vi "Text.vi"(4 "text color(black)":u32(colorbox), 5 "[user-specified font]":T1={"Font Name:"="", "Size"=12, "Strikeout?"=FALSE, "Italic?"=FALSE, "Underline?"=FALSE, "Outline?"=FALSE, "Shadow?"=FALSE, "Bold?"=FALSE}, 6 "alignment(left, top)":T2, 7 "text":string, 8 "error in (no error)":errorcluster, 9 "origin":cluster{"x":i16, "y":i16}, 10 "picture":picture) -> (0 "error out":errorcluster, 2 "new picture":picture)   [LabVIEW 2020, in "lv_icon.lvlib"]
doc: "Add text to a given glyph."
uses:
  <vilib>/LabVIEW Icon API/lv_icon/lv_icon.lvlib
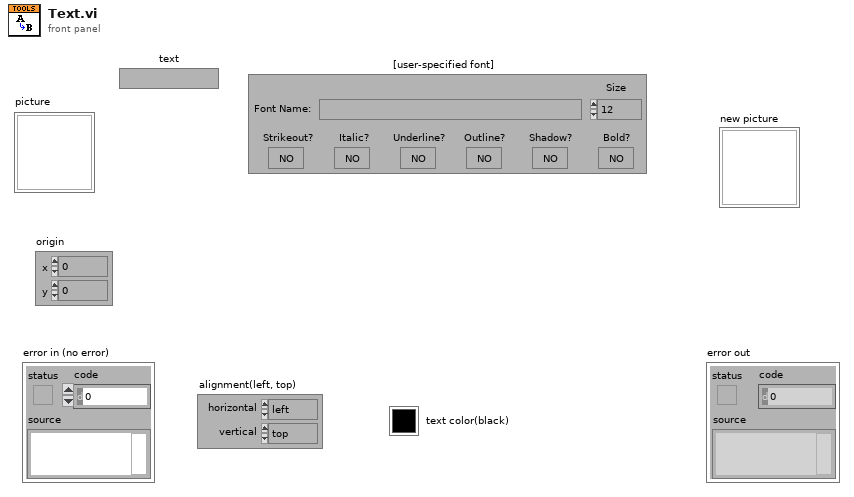
[diagram p1: front panel]
types:
  T1 = cluster{"Font Name:":string, "Size":i16, "Strikeout?":bool, "Italic?":bool, "Underline?":bool, "Outline?":bool, "Shadow?":bool, "Bold?":bool}
  T2 = cluster{"horizontal":enum16{"left", "center", "right"}, "vertical":enum16{"top", "center", "bottom"}}
  T3 = enum16{"User-specified Font", "Application Font", "System Font", "Dialog Font"}
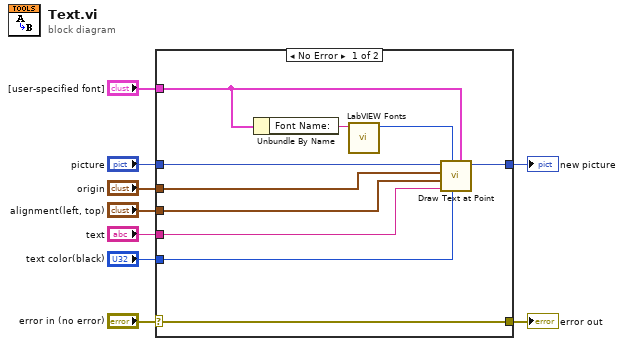
[diagram p0: block diagram]
diagram:
  n1 = case shown="No Error" "error in (no error)" {
    selector: "error in (no error)" -> [w19 w20]
    tunnel: [w19 w20] -> w8
    tunnel: [w18 _] -> w1
    tunnel: "picture" -> [w17 _]
    tunnel: "origin" -> [w16 _]
    tunnel: "alignment(left, top)" -> [w15 _]
    tunnel: "text" -> [w14 _]
    tunnel: "[user-specified font]" -> [w12 _]
    tunnel: "text color(black)" -> [w13 _]
    frame No Error {
      n2 = Unbundle By Name(w12) -> ("Font Name:"=w11:string)
      n3 = call <vilib>:"LabVIEW Fonts.vi"("Font"=w11) -> ("Desired font"=w10:T3)  [unwired: 10 out]
      n4 = call <vilib>:"Draw Text at Point.vi"("[user-specified font]"=w12, "text color(black)"=w13, "desired font(Application)"=w10, "text"=w14, "alignment(left, top)"=w15, "origin"=w16, "picture"=w17) -> ("new picture"=w18:picture)  [unwired: 2 in, 2 out]
    }
    frame Error {
    }
  }
  "error out" <- w8
  "new picture" <- w1
